vi "Write Debug Information.vi"(6 "Timeout Property found?":bool, 7 "Update Property Found?":bool, 8 "error in":errorcluster, 10 "Tags to write":i32, 11 "Tags to read":i32) -> (0 "error out":errorcluster, 3 "Debug String":string)   [LabVIEW 2011, in "Ethernet IP Custom Device Custom Device.lvlib"]
doc: "Creates some simple debugging information and status information that we can either save to disk or print out on the console or display."
uses:
  Ethernet IP Custom Device Custom Device.lvlib
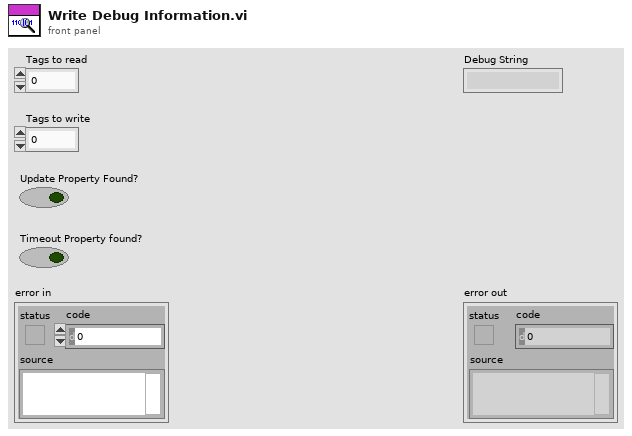
[diagram p1: front panel]
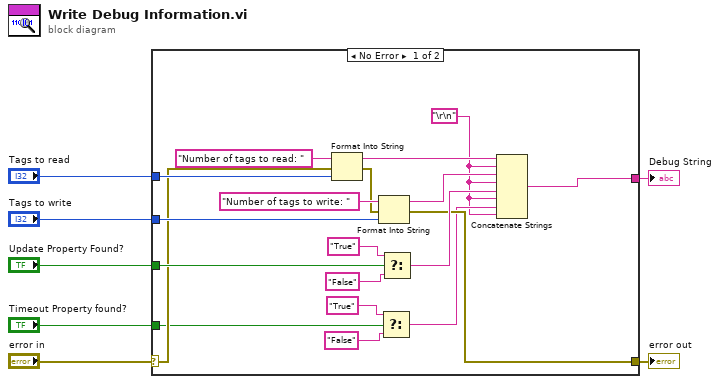
[diagram p0: block diagram]
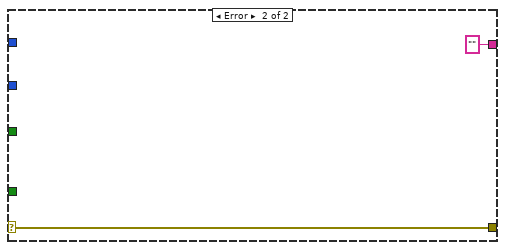
[diagram p2: hidden frame]
diagram:
  n1 = case shown="No Error" "error in" {
    selector: "error in" -> [w16 w28]
    tunnel: "Update Property Found?" -> [w26 _]
    tunnel: "Tags to write" -> [w25 _]
    tunnel: "Tags to read" -> [w24 _]
    tunnel: [w14 w28] -> w3
    tunnel: [w13 ""] -> w2
    tunnel: "Timeout Property found?" -> [w10 _]
    frame No Error {
      w8 = "\r\n"
      n2 = Format Into String(initial string="Number of tags to read: ", error in=w16, w24) -> (resulting string=w19:string, error out=w15:errorcluster)  [unwired: 1 in]
      n3 = Format Into String(initial string="Number of tags to write: ", error in=w15, w25) -> (resulting string=w18:string, error out=w14:errorcluster)  [unwired: 1 in]
      n4 = Select(t="True", s=w10, f="False") -> (s? t:f=w9:string)
      n5 = Select(t="True", s=w26, f="False") -> (s? t:f=w17:string)
      n6 = Concatenate Strings(w19, w8, w18, w8, w17, w8, w9, w8) -> (w13:string)
    }
    frame Error {
    }
  }
  "error out" <- w3
  "Debug String" <- w2
